vi "Read Key Value Boolean.vi"(7 "Section Name":string, 8 "error in (no error)":errorcluster, 9 "Default":bool, 10 "Key Name":string, 11 "ODBC-Interface in":refnum<class "ODBC-Interface.lvclass">) -> (0 "error out":errorcluster, 1 "Value":bool, 2 "found":bool, 3 "ODBC-Interface out":refnum<class "ODBC-Interface.lvclass">)   [LabVIEW 2014, in "DB-Configuration.lvlib" / "ODBC-Interface.lvclass"]
doc: "Read boolean key value."
uses:
  ODBC-Interface.lvclass
  <vilib>/addons/database/_DB Variant To Data/Database Variant To Data.xnode
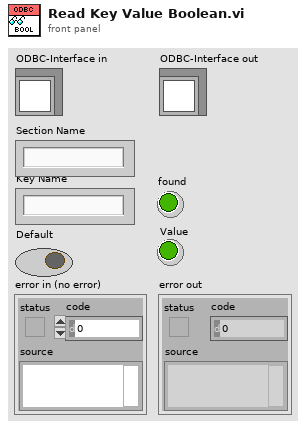
[diagram p1: front panel]
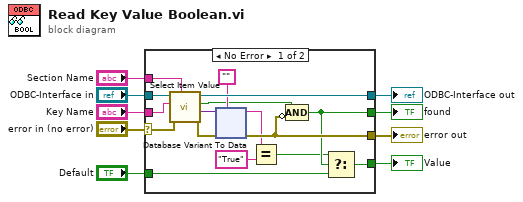
[diagram p0: block diagram]
diagram:
  n1 = case shown="No Error" "error in (no error)" {
    selector: "error in (no error)" -> [w10 w59]
    tunnel: "ODBC-Interface in" -> [w25 w60]
    tunnel: [w24 w60] -> w8
    tunnel: "Section Name" -> [w23 _]
    tunnel: "Key Name" -> [w22 _]
    tunnel: [w17 w59] -> w5
    tunnel: [w15 _] -> w4
    tunnel: [w12 w58] -> w3
    tunnel: "Default" -> [w11 w58]
    frame No Error {
      n2 = call-dynamic "Select Item Value.vi"("Section Name"=w23, "error in (no error)"=w10, "Key Name"=w22, "ODBC-Interface in"=w25) -> ("error out"=w20:errorcluster, "Value"=w21:variant, "found"=w18:bool, "ODBC-Interface out"=w24:refnum<class "ODBC-Interface.lvclass">)  [unwired: 4 in]
      n3 = xnode "Database Variant To Data"("database variant"=w21, "error in (no error)"=w20, "type"="") -> ("data"=w14:string, "error out"=w17:errorcluster)
      n4 = Equal?(x=w14, y="True") -> (x = y?=w13:bool)
      n5 = Compound Arithmetic op=AND(w18, invert w17) -> (w15:bool)
      n6 = Select(t=w13, s=w15, f=w11) -> (s? t:f=w12:bool)
    }
    frame Error {
    }
  }
  "error out" <- w5
  "ODBC-Interface out" <- w8
  "Value" <- w3
  "found" <- w4
